vi "B_ReadProperty.vi"(8 "Error In":errorcluster, 11 "reference in":refnum<class "BaseTemplate_4x4x4.lvclass">) -> (0 "Error Out":errorcluster, 2 "property":dbl, 3 "reference out":refnum<class "BaseTemplate_4x4x4.lvclass">)   [LabVIEW 2020]
uses:
  <resource>/Framework/Providers/Open_GDS/ClassProviders/Provider_EndevoGOOP300/Templates/BaseTemplate_4x4x4/BaseTemplate_4x4x4.lvclass
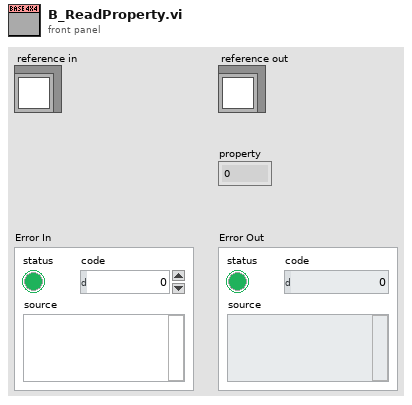
[diagram p1: front panel]
types:
  T1 = typedef "BaseTemplate_4x4x4.lvclass/ObjectAttributes.ctl" = cluster{"Attribute1":dbl}
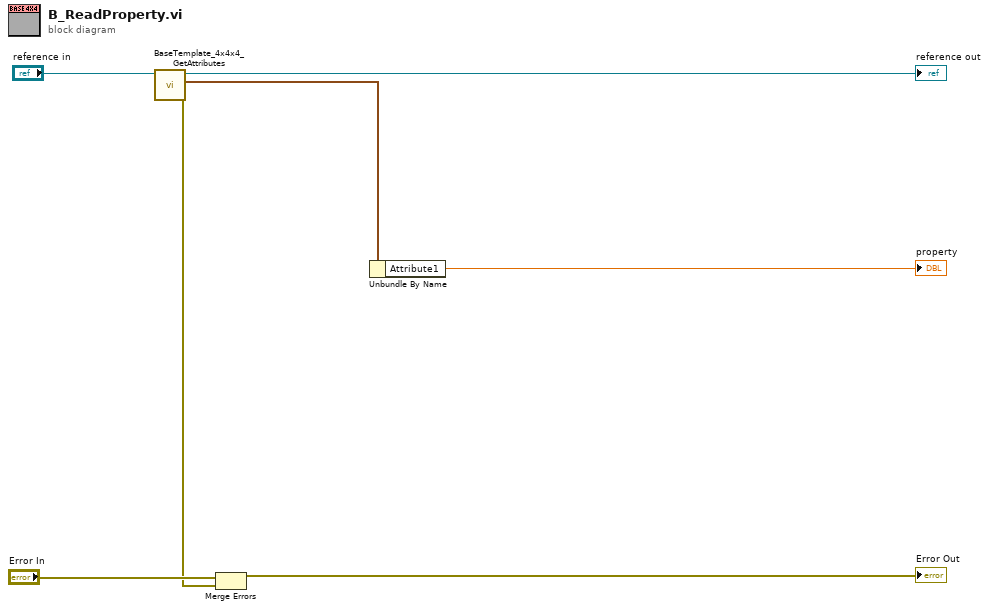
[diagram p0: block diagram]
diagram:
  n1 = call <resource>:"BaseTemplate_4x4x4_GetAttributes.vi"("reference in"="reference in") -> ("error out"=w2:errorcluster, "Attributes"=w4:T1, "reference out"=→"reference out":refnum<class "BaseTemplate_4x4x4.lvclass">)  [unwired: 7 in, 1 out]
  n2 = Merge Errors("Error In", w2) -> (→"Error Out":errorcluster)
  n3 = Unbundle By Name(w4) -> ("Attribute1"=→"property":dbl)
